vi "SVFA Spectrum Peak Search (1 Ch).vi"(0 "spectrum":cluster{"x0":dbl, "dx":dbl, "magnitude":dbl[]} {"magnitude" format="%.2f"; "dx" format="%.2f"; "x0" format="%.2f"}, 1 "peak search settings":T7={"single/multiple"=enum."Multiple Peaks", "threshold"=inf} {"threshold" format="%.2f"}, 4 "spectrum info in":T1={"channel name"="", "description"="", "x-axis units"=0, "spectral info"={"spectrum type"=enum."Power [Magnitude^2]", "linear/dB"=enum."linear", "window"=0, "window size"=0, "FFT size"=0}, "engineering units"=0, "custom label"="", "dB reference [EU]"=0.0, "peak units"=enum."rms", "weighting filter"=0, "spectral density?"=FALSE, "unit label"="", "spectrum skewed?"=FALSE, "complimentary spectrum units"=enum."none"} {"x-axis units" items=["Time (s)"=0, "Frequency-CB (Hz)"=1, "Frequency-CPB (Hz)"=1248, "Frequency-Arbitrary (Hz)"=2357, "Quefrency (s)"=2, "Revolutions (rev)"=3, "Order"=4, "Speed (RPM)"=11, "Speed (rad/s)"=21, "Index"=65535]; "weighting filter" items=["Linear", "A-weighting", "B-weighting", "C-weighting", "ITU-R 468-4", "Dolby", "CCITT", "C-message", "Wb", "Wc", "Wd", "We", "Wf", "Wh", "Wj", "Wk", "Wm", "AES17 20 kHz lowpass", "AES17 40 kHz lowpass", "AES17 20 kHz highpass", "AES17 40 kHz highpass"]; "dB reference [EU]" format="%.2f"; "engineering units" items=["custom..."=0, "V"=1, "A"=21, "C"=30, "pC"=31, "s"=32, "-"=29, "Pa"=2, "N"=20, "g"=3, "m/s^2"=4, "m/s"=5, "m"=6, "mm/s"=12, "mm"=13, "micron/s"=14, "micron"=15, "in/s^2"=7, "in/s"=8, "in"=9, "mil/s"=10, "mil"=11, "rad/s^2"=16, "rad/s"=17, "rad"=18, "deg/s^2"=26, "deg/s"=27, "deg"=28, "RPM"=22, "cycle/s^2"=23, "Hz"=24, "cycle"=25, "strain"=19]; "spectral info"."window" items=["None "=0, "Hanning"=1, "Hamming"=2, "Blackman-Harris"=3, "Exact Blackman"=4, "Blackman"=5, "Flat Top"=6, "4 Term B-Harris "=7, "7 Term B-Harris"=8, "Low Sidelobe"=9, "Force - Exponential"=10, "Gaussian"=62]}, 5 "error in (no error)":errorcluster) -> (14 "peaks":cluster{"freq. or order":dbl, "value":dbl}[](array[cluster]) {"value" format="%.2f"; "freq. or order" format="%.2f"}, 15 "number of peaks":i32, 16 "unit label":string, 18 "spectrum info out":T1={"channel name"="", "description"="", "x-axis units"=0, "spectral info"={"spectrum type"=enum."Power [Magnitude^2]", "linear/dB"=enum."linear", "window"=0, "window size"=0, "FFT size"=0}, "engineering units"=0, "custom label"="", "dB reference [EU]"=0.0, "peak units"=enum."rms", "weighting filter"=0, "spectral density?"=FALSE, "unit label"="", "spectrum skewed?"=FALSE, "complimentary spectrum units"=enum."none"} {"x-axis units" items=["Time (s)"=0, "Frequency-CB (Hz)"=1, "Frequency-CPB (Hz)"=1248, "Frequency-Arbitrary (Hz)"=2357, "Quefrency (s)"=2, "Revolutions (rev)"=3, "Order"=4, "Speed (RPM)"=11, "Speed (rad/s)"=21, "Index"=65535]; "weighting filter" items=["Linear", "A-weighting", "B-weighting", "C-weighting", "ITU-R 468-4", "Dolby", "CCITT", "C-message", "Wb", "Wc", "Wd", "We", "Wf", "Wh", "Wj", "Wk", "Wm", "AES17 20 kHz lowpass", "AES17 40 kHz lowpass", "AES17 20 kHz highpass", "AES17 40 kHz highpass"]; "dB reference [EU]" format="%.2f"; "engineering units" items=["custom..."=0, "V"=1, "A"=21, "C"=30, "pC"=31, "s"=32, "-"=29, "Pa"=2, "N"=20, "g"=3, "m/s^2"=4, "m/s"=5, "m"=6, "mm/s"=12, "mm"=13, "micron/s"=14, "micron"=15, "in/s^2"=7, "in/s"=8, "in"=9, "mil/s"=10, "mil"=11, "rad/s^2"=16, "rad/s"=17, "rad"=18, "deg/s^2"=26, "deg/s"=27, "deg"=28, "RPM"=22, "cycle/s^2"=23, "Hz"=24, "cycle"=25, "strain"=19]; "spectral info"."window" items=["None "=0, "Hanning"=1, "Hamming"=2, "Blackman-Harris"=3, "Exact Blackman"=4, "Blackman"=5, "Flat Top"=6, "4 Term B-Harris "=7, "7 Term B-Harris"=8, "Low Sidelobe"=9, "Force - Exponential"=10, "Gaussian"=62]}, 19 "error out":errorcluster)   [LabVIEW 2017]
doc: "Performs a peak search on a spectrum or spectra. The spectrum or spectra can be in either the frequency domain or the order domain. Detects single or multiple peaks in Power, PSD, and COP spectra. Wire data to the <B>spectrum</B> input to determine the polymorphic instance to use or manually select the instance."
uses:
  <vilib>/addons/_NISVFA/_Shared subVIs/Controls/svc_Spectrum Info.ctl
  <vilib>/addons/_NISVFA/_Shared subVIs/Controls/svc_X-Axis Units.ctl
  <vilib>/addons/_NISVFA/_Shared subVIs/Controls/svc_Spectrum Type.ctl
  <vilib>/addons/_NISVFA/_Shared subVIs/Controls/svc_Engineering Units Text Ring.ctl
  <vilib>/addons/_NISVFA/_Shared subVIs/Controls/svc_Weighting Filter Text Ring.ctl
  <vilib>/addons/_NISVFA/_Shared subVIs/Controls/svc_Complimentary Spectrum Units.ctl
  <vilib>/addons/_NISVFA/_Spectrum Processing/subVIs/svfa_Peak Rough Search Indices.vi
  <vilib>/addons/_NISVFA/_Shared subVIs/Common/svc_Get Weighting Enum and Labels.vi
  <vilib>/addons/_NISVFA/_Shared subVIs/Common/svc_Unit Label Lexical Class.vi
  <vilib>/addons/_NISVFA/_Shared subVIs/Common/svc_Engineering Units to Unit Label.vi
  <vilib>/addons/_NISVFA/_Shared subVIs/Common/svc_Format Value (DBL).vi
  <vilib>/addons/_NISVFA/_Spectrum Processing/subVIs/svfa_Three Finger Peak Search.vi
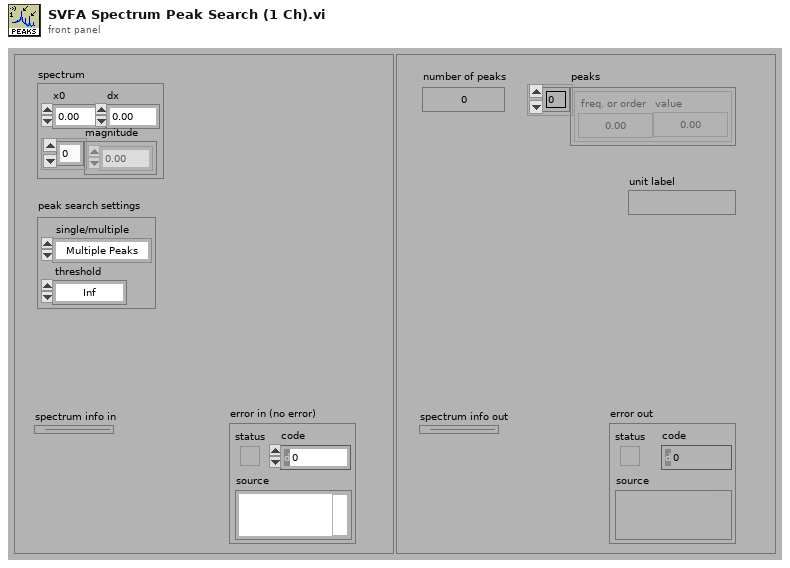
[diagram p1: front panel]
types:
  T1 = typedef "svc_Spectrum Info.ctl" = cluster{"channel name":string, "description":string, "x-axis units":T2, "spectral info":cluster{"spectrum type":T3, "linear/dB":enum16{"linear", "dB"}, "window":u16, "window size":i32, "FFT size":i32}, "engineering units":T4, "custom label":string, "dB reference [EU]":dbl, "peak units":enum16{"rms", "peak", "peak-peak"}, "weighting filter":T5, "spectral density?":bool, "unit label":string, "spectrum skewed?":bool, "complimentary spectrum units":T6}
  T2 = typedef "svc_X-Axis Units.ctl" = u16
  T3 = typedef "svc_Spectrum Type.ctl" = enum16{"FFT Spectrum [complex]", "Amplitude [Magnitude]", "Power [Magnitude^2]", "Cross Spectrum [complex]", "Frequency Response [Complex]"}
  T4 = typedef "svc_Engineering Units Text Ring.ctl" = u16
  T5 = typedef "svc_Weighting Filter Text Ring.ctl" = u16
  T6 = typedef "svc_Complimentary Spectrum Units.ctl" = enum16{"none", "radians", "degrees", "cycles", "imaginary"}
  T7 = cluster{"single/multiple":enum16{"Multiple Peaks", "Single Max Peak"}, "threshold":dbl}
  T8 = cluster{"spectrum type":T3, "linear/dB":enum16{"linear", "dB"}, "window":u16, "window size":i32, "FFT size":i32}
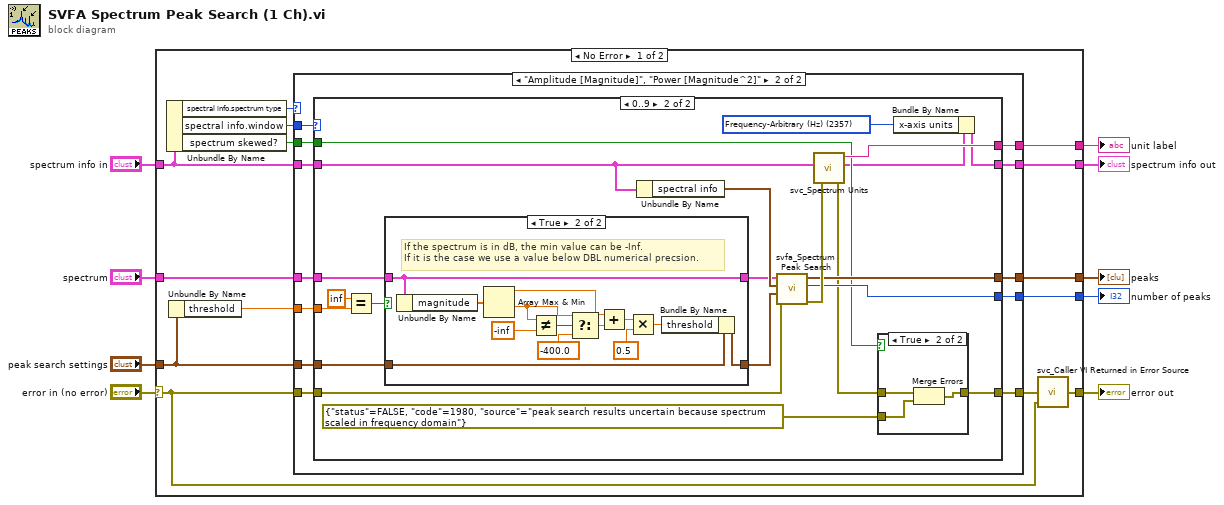
[diagram p0: block diagram]
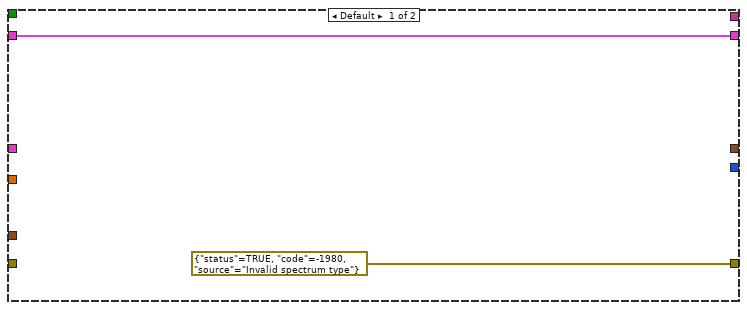
[diagram p2: hidden frame]
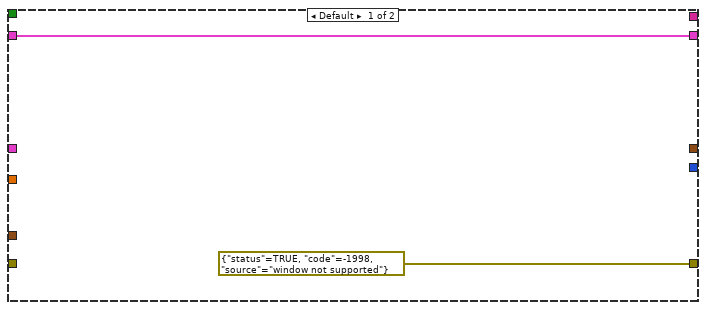
[diagram p3: hidden frame]
diagram:
  n1 = case shown="No Error" "error in (no error)" {
    selector: "error in (no error)" -> [w15 w81]
    tunnel: "spectrum" -> [w19 _]
    tunnel: "peak search settings" -> [w10 _]
    tunnel: [w23 _] -> w7
    tunnel: [w22 _] -> w6
    tunnel: [w20 w81] -> w5
    tunnel: [w21 _] -> w4
    tunnel: "spectrum info in" -> [w18 w80]
    tunnel: [w11 w80] -> w1
    frame No Error {
      n2 = Unbundle By Name(w18) -> ("spectral info.spectrum type"=w17:T3, "spectral info.window"=w16:u16, "spectrum skewed?"=w12:bool)
      n3 = Unbundle By Name(w10) -> ("threshold"=w13:dbl)
      n4 = case shown="\"Amplitude [Magnitude]\", \"Power [Magnitude^2]\"" w17 {
        tunnel: [_ w37] -> w23
        tunnel: [_ w36] -> w22
        tunnel: [errorcluster {"status"=TRUE, "code"=-1980, "source"="Invalid spectrum type"} ("error out") w35] -> w14
        tunnel: [_ w34] -> w21
        tunnel: w19 -> [_ w33]
        tunnel: w15 -> [_ w32]
        tunnel: w18 -> [w24 w31]
        tunnel: w16 -> [_ w30]
        tunnel: w10 -> [_ w29]
        tunnel: w13 -> [_ w28]
        tunnel: w12 -> [_ w27]
        tunnel: [w24 w26] -> w11
        frame Default {
        }
        frame "Amplitude [Magnitude]", "Power [Magnitude^2]" {
          n5 = case shown="0..9" w30 {
            tunnel: [_ w56] -> w37
            tunnel: [_ w57] -> w36
            tunnel: [errorcluster {"status"=TRUE, "code"=-1998, "source"="window not supported"} ("error out") w44] -> w35
            tunnel: [_ w60] -> w34
            tunnel: w33 -> [_ w54]
            tunnel: w32 -> [_ w47]
            tunnel: w31 -> [w38 w55]
            tunnel: w29 -> [_ w51]
            tunnel: w28 -> [_ w49]
            tunnel: w27 -> [_ w46]
            tunnel: [w38 w40] -> w26
            frame Default {
            }
            frame 0..9 {
              w42 = T2 2357 items=["Time (s)"=0, "Frequency-CB (Hz)"=1, "Frequency-CPB (Hz)"=1248, "Frequency-Arbitrary (Hz)"=2357, "Quefrency (s)"=2, "Revolutions (rev)"=3, "Order"=4, "Speed (RPM)"=11, "Speed (rad/s)"=21, "Critical Band"=31, "Critical Band Rate (Bark)"=32, "Index"=65535] ("x-axis units")
              n6 = Equal?(x=inf ("y"), y=w49) -> (x = y?=w48:bool)
              n7 = case shown="True" w48 {
                tunnel: w54 -> [w66 w78]
                tunnel: w51 -> [w65 w79]
                tunnel: [w65 w67] -> w52
                tunnel: [w66 w78] -> w53
                frame False {
                }
                frame True {
                  # "If the spectrum is in dB, the min value can be -Inf.\nIf it is the case we use a value below DBL numerical precsion."
                  n8 = Unbundle By Name(w78) -> ("magnitude"=w77:dbl[])
                  n9 = Array Max & Min(array=w77) -> (max value=w76:dbl, min value=w70:dbl)  [unwired: 2 out]
                  n10 = Not Equal?(x=w70, y=-inf) -> (x != y?=w72:bool)
                  n11 = Select(t=w70, s=w72, f=-400.0 ("y")) -> (s? t:f=w69:dbl)
                  n12 = Add(x=w76, y=w69) -> (x+y=w75:dbl)
                  n13 = Multiply(x=w75, y=0.5) -> (x*y=w73:dbl)
                  n14 = Bundle By Name(cluster=w79, "threshold"=w73) -> (w67:T7)
                }
              }
              n15 = Unbundle By Name(w55) -> ("spectral info"=w59:T8)
              n16 = call <vilib>:"svfa_Spectrum Peak Search.vi"("error in (no error)"=w47, "peak search settings"=w52, "spectral info"=w59, "spectrum"=w53) -> ("error out"=w58:errorcluster, "# of peaks"=w57:i32, "peaks"=w56:cluster{"frequency":dbl, "Value":dbl}[])  [unwired: 5 in]
              n17 = call <vilib>:"svc_Spectrum Units.vi"("error in (no error)"=w58, "spectrum info in"=w55) -> ("error out"=w45:errorcluster, "spectrum info out"=w41:T1, "unit label"=w60:string)  [unwired: 2 in, 1 out]
              n18 = case shown="True" w46 {
                tunnel: [w61 w63] -> w44
                tunnel: w45 -> [w61 w64]
                tunnel: errorcluster {"status"=FALSE, "code"=1980, "source"="peak search results uncertain because spectrum scaled in frequency domain"} ("error in 2 (no error)") -> [_ w62]
                frame False {
                }
                frame True {
                  n19 = Merge Errors(w64, w62) -> (w63:errorcluster)
                }
              }
              n20 = Bundle By Name(cluster=w41, "x-axis units"=w42) -> (w40:T1)
            }
          }
        }
      }
      n21 = call <vilib>:"svc_Caller VI Returned in Error Source.vi"("warning input to caller"=w15, "error in (no error)"=w14) -> ("error out"=w20:errorcluster)  [unwired: 3 in]
    }
    frame Error {
    }
  }
  "error out" <- w5
  "peaks" <- w7
  "number of peaks" <- w6
  "unit label" <- w4
  "spectrum info out" <- w1
